vi "obtainSALLVFunctionReferences.vi"(8 "error in (no error)":errorcluster, 11 "timestamp in":refnum<class "timestamp.lvclass">) -> (0 "error out":errorcluster, 3 "timestamp out":refnum<class "timestamp.lvclass">)   [LabVIEW 2016, in "SALLV_AtDome_Messaging.lvlib" / "timestamp.lvclass"]
uses:
  timestamp.lvclass
  home/andres/ts_AtDome/SALTopic/SALTopic/SALTopic.lvclass
  timestamp.lvclass/timestamp.ctl
  SALTopic/SALTelemetry/SALTelemetry.lvclass
  SALTopic/SALTopic/SALTopic.lvclass
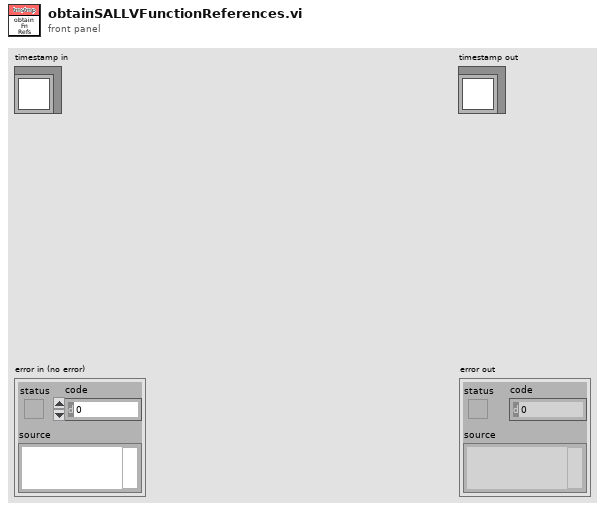
[diagram p1: front panel]
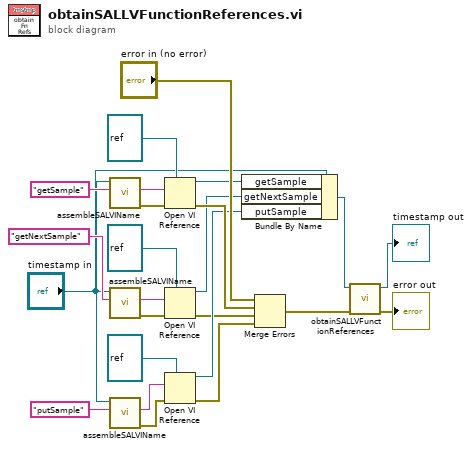
[diagram p0: block diagram]
diagram:
  n1 = call "assembleSALVIName.vi"("topicKey"="getSample" ("commandKey"), "SALTopic in"="timestamp in") -> ("error out"=w23:errorcluster, "viPath"=w24:string)  [unwired: 7 in, 1 out]
  n2 = call "assembleSALVIName.vi"("topicKey"="getNextSample" ("commandKey"), "SALTopic in"="timestamp in") -> ("error out"=w9:errorcluster, "viPath"=w8:string)  [unwired: 7 in, 1 out]
  n3 = call "assembleSALVIName.vi"("topicKey"="putSample" ("commandKey"), "SALTopic in"="timestamp in") -> ("error out"=w21:errorcluster, "viPath"=w22:string)  [unwired: 7 in, 1 out]
  n4 = Open VI Reference(type specifier VI Refnum (for type only)=refnum<vi> refnum ("reference"), vi path=w24, error in (no error)=w23) -> (vi reference=w13:refnum<vi>, error out=w15:errorcluster)  [unwired: 3 in]
  n5 = Open VI Reference(type specifier VI Refnum (for type only)=refnum<vi> refnum ("reference"), vi path=w8, error in (no error)=w9) -> (vi reference=w7:refnum<vi>, error out=w6:errorcluster)  [unwired: 3 in]
  n6 = Open VI Reference(type specifier VI Refnum (for type only)=refnum<vi> refnum ("reference"), vi path=w22, error in (no error)=w21) -> (vi reference=w12:refnum<vi>, error out=w14:errorcluster)  [unwired: 3 in]
  n7 = Bundle By Name(cluster="timestamp in", "getSample"=w13, "getNextSample"=w7, "putSample"=w12) -> (w4:refnum<class "timestamp.lvclass">)
  n8 = Merge Errors("error in (no error)", w15, w6, w14) -> (w2:errorcluster)
  n9 = call-parent "obtainSALLVFunctionReferences.vi"("error in (no error)"=w2, "SALTelemetry in"=w4) -> ("error out"=→"error out":errorcluster, "SALTelemetry out"=→"timestamp out":refnum<class "timestamp.lvclass">)  [unwired: 8 in]
